vi "Proj_num.vi"(1 "Update Proj Num-Name?":bool) -> (0 "ProjectNumber":string)   [LabVIEW 2022 SP3]
uses:
  Setup_Filetype.ctl
  Globals/Preference_global.vi
panel:
  # "Looks for file Current_Project.txt in current General preferences and uses it as starting value in interactive ProjNum prompt.\nIF the file contains s string in the form:\n\"FixedProject=WXYZ\" then WXYZ will be used as the Project Name without prompting (Intended for use with metadata servers, for instance)"
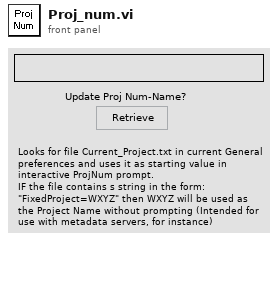
[diagram p1: front panel]
types:
  T1 = typedef "Setup_Filetype.ctl" = enum16{"Measurement Setups", "Calibration Setups", "General", "Results File Plotter Setups", "Speed Calib Tweaks"}
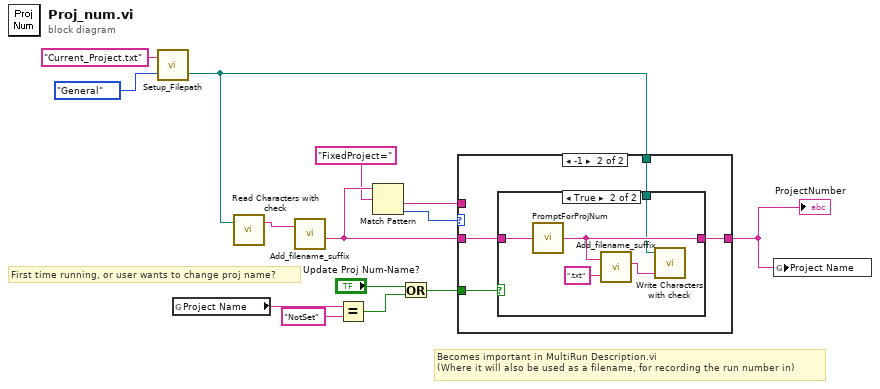
[diagram p0: block diagram]
diagram:
  # "Becomes important in MultiRun Description.vi\n(Where it will also be used as a filename, for recording the run number in)"
  # "First time running, or user wants to change proj name?"
  n1 = call "Setup_Filepath.vi"("Setup File Type"=Setup_Filetype."General", "Filename in"="Current_Project.txt") -> ("Filename Out"=w2:path)  [unwired: 1 out]
  n2 = global read "Preference_global.vi" "Project Name"() -> (w12:string)
  n3 = call "Read Characters with check.vi"("file (use dialog)"=w2) -> ("Read String"=w1:string)  [unwired: 1 in, 1 out]
  n4 = call "Add_filename_suffix.vi"("Filename"=w1) -> ("Base name"=w7:string)  [unwired: 1 in, 3 out]
  n5 = Equal?(x=w12, y="NotSet") -> (x = y?=w11:bool)
  n6 = Match Pattern(string=w7, regular expression="FixedProject=") -> (after substring=w4:string, offset past match=w5:i32)  [unwired: 1 in, 2 out]
  n7 = Or(x="Update Proj Num-Name?", y=w11) -> (x .or. y?=w13:bool)
  n8 = case shown="-1" w5 {
    tunnel: w13 -> [_ w19]
    tunnel: [w15 w18] -> w3
    tunnel: w7 -> [_ w17]
    tunnel: w4 -> [w15 _]
    tunnel: w2 -> [_ w16]
    frame 0, Default {
    }
    frame -1 {
      n9 = case shown="True" w19 {
        tunnel: [w20 w23] -> w18
        tunnel: w17 -> [w20 w25]
        tunnel: w16 -> [_ w22]
        frame False {
        }
        frame True {
          n10 = call "PromptForProjNum.vi"("project"=w25) -> ("ProjectNumber OUT"=w23:string)
          n11 = call "Add_filename_suffix.vi"("Filename"=w23, "Suffix to add"=".txt") -> ("Filename out"=w21:string)  [unwired: 3 out]
          n12 = call "Write Characters with check.vi"("String to Write"=w21, "file (use dialog)"=w22) -> ()  [unwired: 2 in, 1 out]
        }
      }
    }
  }
  "ProjectNumber" <- w3
  n13 = global write "Preference_global.vi" "Project Name"(w3) -> ()
